vi "Exercise 7.3_Answer.vi"() -> ()   [LabVIEW 2020]
uses:
  7.3 States.ctl
panel:
  out "Button References":refnum<vi>[](array[refnum])
  out "Locked/Unlocked":bool
  in  "Clear":bool
  out "Code Entered":string
  in  "Enter":bool
  in  "Button 9":bool
  in  "Button 8":bool
  in  "Button 7":bool
  in  "Button 6":bool
  in  "Button 5":bool
  in  "Button 4":bool
  in  "Button 3":bool
  in  "Button 2":bool
  in  "Button 1":bool
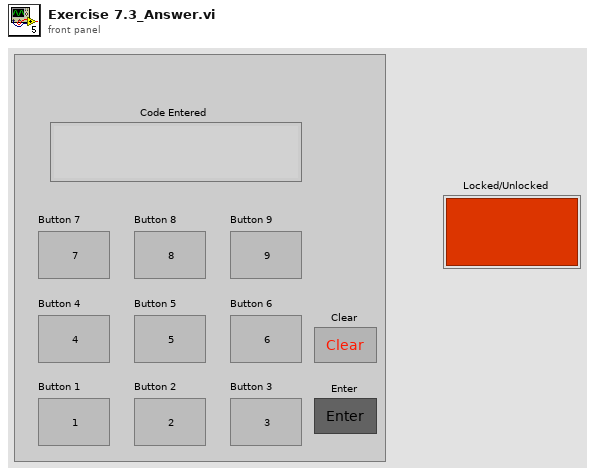
[diagram p1: front panel]
types:
  T1 = typedef "7.3 States.ctl" = enum16{"Initialize", "Button Was Pressed", "Wait", "Clear", "Check Code"}
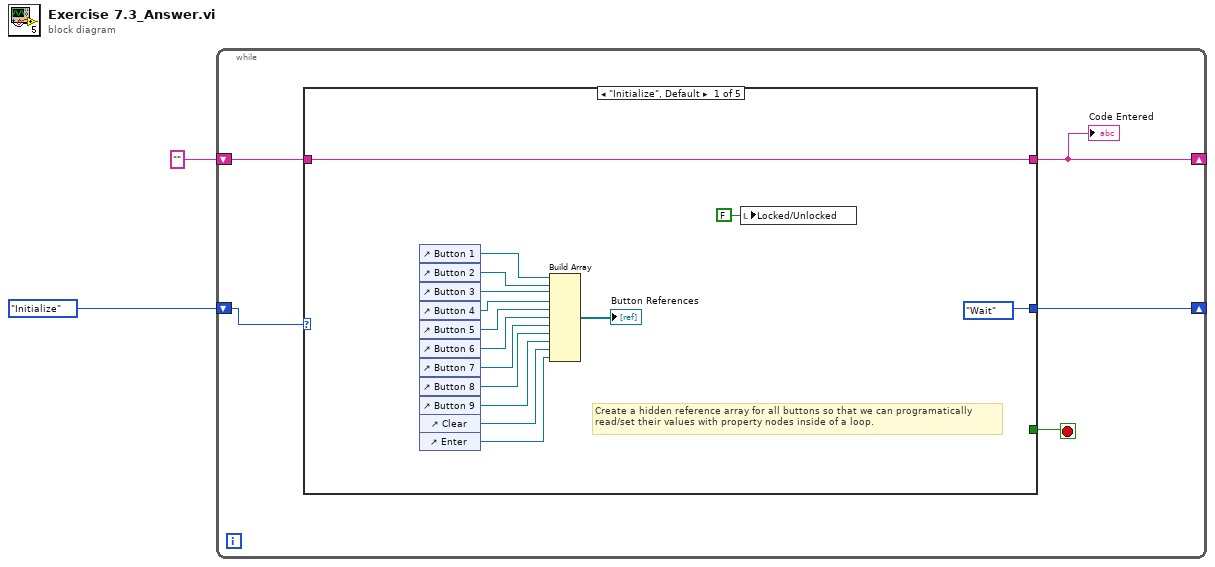
[diagram p0: block diagram]
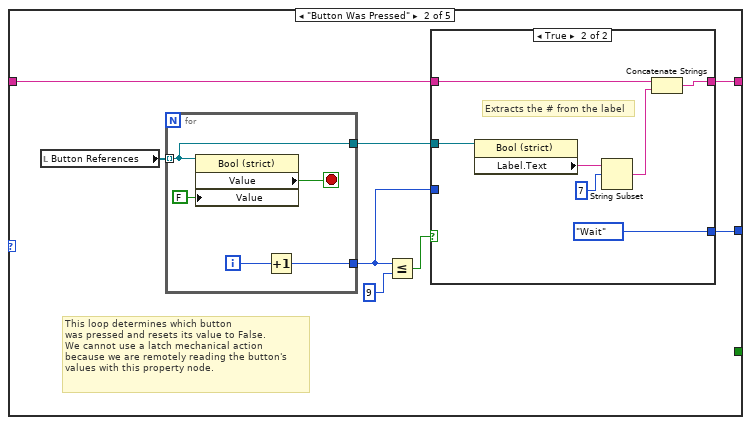
[diagram p2: hidden frame]
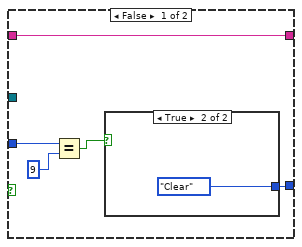
[diagram p3: hidden frame]
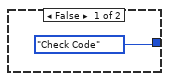
[diagram p4: hidden frame]
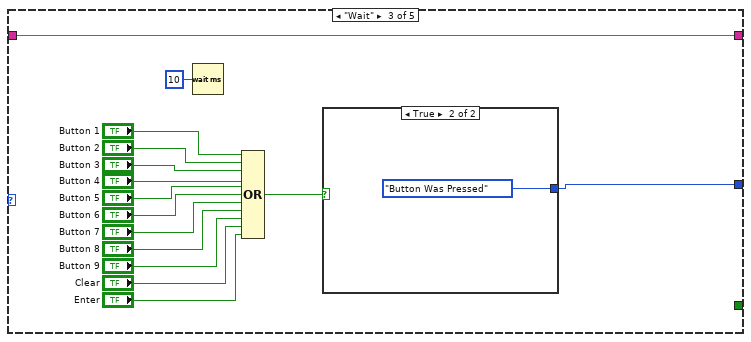
[diagram p5: hidden frame]
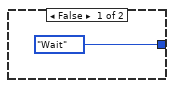
[diagram p6: hidden frame]
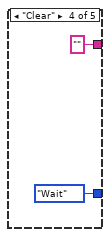
[diagram p7: hidden frame]
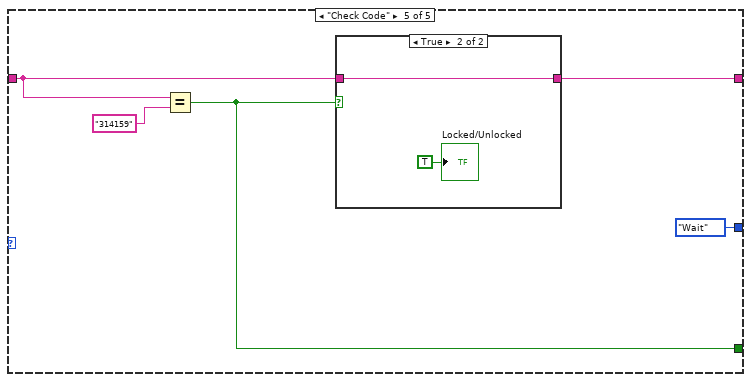
[diagram p8: hidden frame]
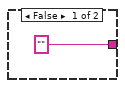
[diagram p9: hidden frame]
diagram:
  n1 = while {
    shift-right: [w6] -> _
    shift-left: 7.3_States."Initialize" -> [w7]
    shift-right: [w4] -> _
    shift-left: "" -> [w5]
    stop <- w3 stop-if-true
    n2 = case shown="\"Initialize\", Default" w7 {
      tunnel: [7.3_States."Wait" w24 w53 7.3_States."Wait" 7.3_States."Wait"] -> w6
      tunnel: w5 -> [w11 w26 w50 _ w71]
      tunnel: [w11 w25 w50 "" w70] -> w4
      tunnel: [_ _ _ _ w72] -> w3
      frame "Initialize", Default {
        # "Create a hidden reference array for all buttons so that we can programatically\nread/set their values with property nodes inside of a loop."
        n3 = control-ref of="Button 1"() -> (w14:refnum<vi>)
        n4 = control-ref of="Button 2"() -> (w15:refnum<vi>)
        n5 = control-ref of="Button 3"() -> (w16:refnum<vi>)
        n6 = control-ref of="Button 4"() -> (w17:refnum<vi>)
        n7 = control-ref of="Button 5"() -> (w18:refnum<vi>)
        n8 = control-ref of="Button 6"() -> (w19:refnum<vi>)
        n9 = control-ref of="Button 7"() -> (w20:refnum<vi>)
        n10 = control-ref of="Button 8"() -> (w21:refnum<vi>)
        n11 = control-ref of="Button 9"() -> (w22:refnum<vi>)
        n12 = control-ref of="Clear"() -> (w10:refnum<vi>)
        n13 = control-ref of="Enter"() -> (w9:refnum<vi>)
        n14 = Build Array(w14, w15, w16, w17, w18, w19, w20, w21, w22, w10, w9) -> (→"Button References":refnum<vi>[])
        n15 = local write "Locked/Unlocked"(FALSE ("Locked/Unlocked")) -> ()
      }
      frame "Button Was Pressed" {
        # "This loop determines which button\nwas pressed and resets its value to False.\nWe cannot use a latch mechanical action\nbecause we are remotely reading the button's \nvalues with this property node."
        n16 = local read "Button References"() -> (w30:refnum<vi>[])
        n17 = for {
          tunnel: w30 -> [w45] mode=indexing
          tunnel: [w47] -> w23
          tunnel: [w45] -> w27
          i -> [w49]
          stop <- w48 stop-if-true
          n18 = property class="Bool (strict)"(reference=w45, "Value"=FALSE) -> ("Value"=w48:bool)  [unwired: 1 in, 2 out]
          n19 = Increment(x=w49) -> (x+1=w47:i32)
        }
        n20 = Less Or Equal?(x=w23, y=9) -> (x <= y?=w28:bool)
        n21 = case shown="True" w28 {
          tunnel: w27 -> [_ w44]
          tunnel: w26 -> [w31 w41]
          tunnel: [w31 w39] -> w25
          tunnel: [w32 7.3_States."Wait"] -> w24
          tunnel: w23 -> [w35 _]
          frame False {
            n22 = Equal?(x=w35, y=9) -> (x = y?=w33:bool)
            n23 = case shown="True" w33 {
              tunnel: [7.3_States."Check Code" 7.3_States."Clear"] -> w32
              frame False {
              }
              frame True {
              }
            }
          }
          frame True {
            # "Extracts the # from the label"
            n24 = property class="Bool (strict)"(reference=w44) -> ("Label.Text"=w43:string)  [unwired: 1 in, 2 out]
            n25 = String Subset(string=w43, offset (0)=7) -> (substring=w40:string)  [unwired: 1 in]
            n26 = Concatenate Strings(w41, w40) -> (w39:string)
          }
        }
      }
      frame "Wait" {
        n27 = Wait (ms)(milliseconds to wait=u32 10) -> ()  [unwired: 1 out]
        n28 = Compound Arithmetic op=OR("Button 1", "Button 2", "Button 3", "Button 4", "Button 5", "Button 6", "Button 7", "Button 8", "Button 9", "Clear", "Enter") -> (w55:bool)
        n29 = case shown="True" w55 {
          tunnel: [7.3_States."Wait" 7.3_States."Button Was Pressed"] -> w53
          frame False {
          }
          frame True {
          }
        }
      }
      frame "Clear" {
      }
      frame "Check Code" {
        n30 = Equal?(x=w71, y="314159") -> (x = y?=w72:bool)
        n31 = case shown="True" w72 {
          tunnel: w71 -> [_ w76]
          tunnel: ["" w76] -> w70
          frame False {
          }
          frame True {
            "Locked/Unlocked" <- TRUE ("Locked/Unlocked")
          }
        }
      }
    }
    "Code Entered" <- w4
  }
